vi "ReadSensorValues_v1.1.vi"(10 "VISA resource name":refnum<visa-resource-name>, 11 "Sensor type":T1) -> ()   [LabVIEW 2012]
uses:
  <vilib>/nican/nicantsk.llb/CAN Interface.ctl
  SensorTypes.ctl
  SensorStates.ctl
  <vilib>/nican/nicantsk.llb/CAN Task Reference.ctl
  <vilib>/nican/nicantsk.llb/CAN Mode.ctl
  globalVariables.vi
  <vilib>/nican/nicantsk.llb/CAN Read Multi Chan Single Samp 1D Dbl.vi
  <instrlib>/Agilent 34970/Agilent 34970.lvlib
panel:
  in  "Sample time reference sensor / s":dbl=0.05
  in  "VISA resource name 2":refnum<visa-resource-name>="USB0::0x0957::0x2007::MY49004365::INSTR"
  in  "Cancel Measurement":bool
  out "new data":bool
  out "running":bool
  out "Sample number":i32
  in  "Interface":T2 items=["CAN0"=0, "CAN1"=1, "CAN2"=2, "CAN3"=3, "CAN4"=4, "CAN5"=5, "CAN6"=6, "CAN7"=7, "CAN8"=8, "CAN9"=9, "CAN10"=10, "CAN11"=11, "CAN12"=12, "CAN13"=13, "CAN14"=14, "CAN15"=15, "CAN16"=16, "CAN17"=17, "CAN18"=18, "CAN19"=19, "CAN20"=20, "CAN21"=21, "CAN22"=22, "CAN23"=23, "CAN24"=24, "CAN25"=25, "CAN26"=26, "CAN27"=27, "CAN28"=28, "CAN29"=29, "CAN30"=30, "CAN31"=31, "CAN32"=32, "CAN33"=33, "CAN34"=34, "CAN35"=35, "CAN36"=36, "CAN37"=37, "CAN38"=38, "CAN39"=39, "CAN40"=40, "CAN41"=41, "CAN42"=42, "CAN43"=43, "CAN44"=44, "CAN45"=45, "CAN46"=46, "CAN47"=47, "CAN48"=48, "CAN49"=49, "CAN50"=50, "CAN51"=51, "CAN52"=52, "CAN53"=53, "CAN54"=54, "CAN55"=55, "CAN56"=56, "CAN57"=57, "CAN58"=58, "CAN59"=59, "CAN60"=60, "CAN61"=61, "CAN62"=62, "CAN63"=63, "MAX default"=64, "CAN256 (Virtual)"=256, "CAN257 (Virtual)"=257]
  out "Error Flag":bool
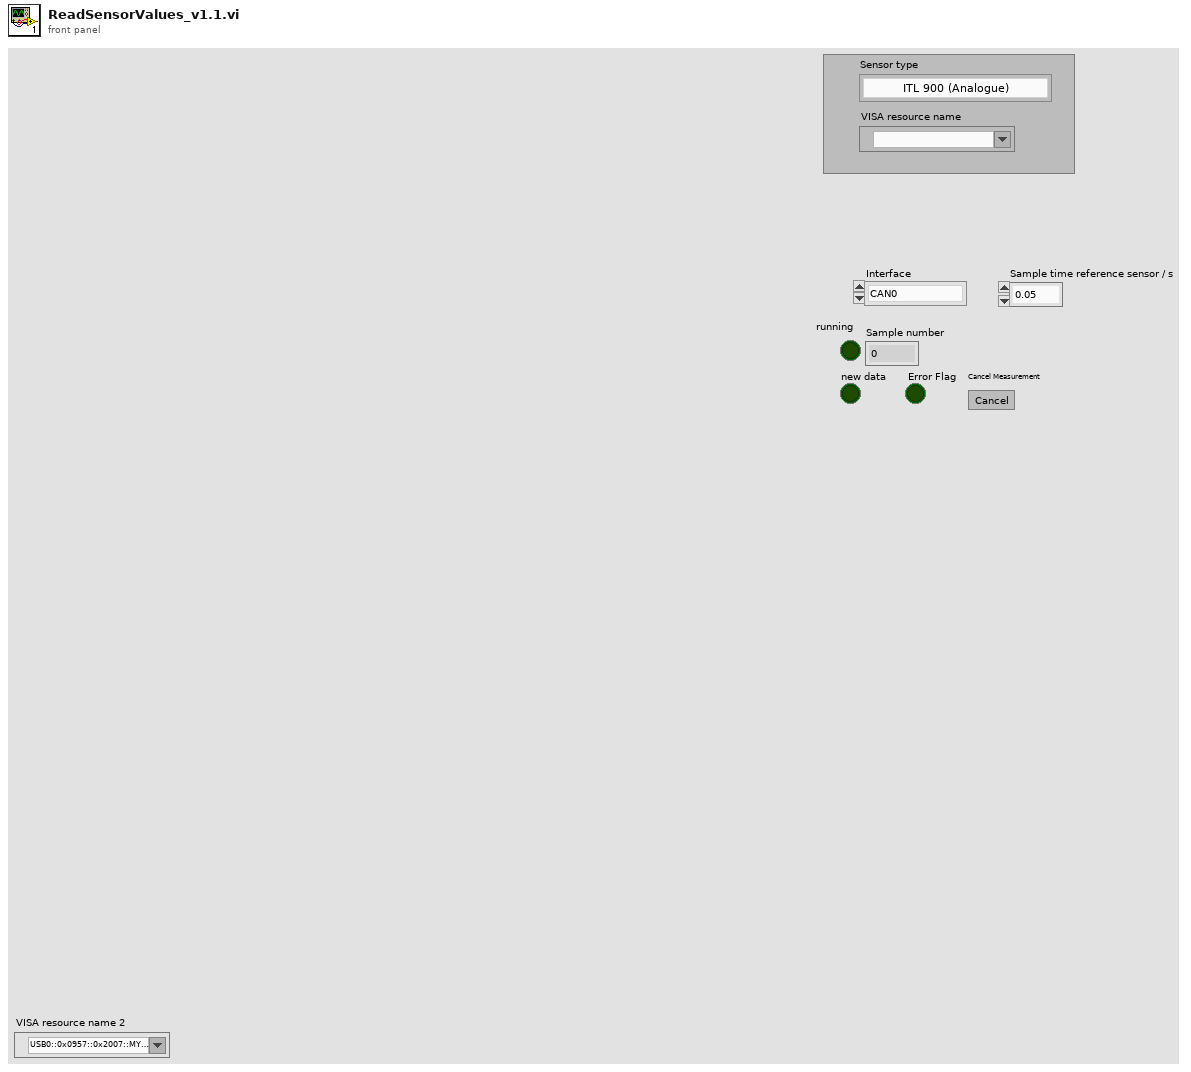
[diagram p1: front panel]
types:
  T1 = typedef "SensorTypes.ctl" = enum16{"ITL 900 (Analogue)", "CAB 300-C SP3 (CAN)", "xyz TODO (PWM)", "xyz TODO (LIN)", "xyz TODO (Analogue)"}
  T2 = typedef "CAN Interface.ctl" = u16
  T3 = typedef "SensorStates.ctl" = enum16{"init", "measure", "terminate"}
  T4 = cluster{"Include Alarm Data F:(No)":bool, "Include Channel # (F:No)":bool, "Include Time (F:No)":bool, "Include Units (F:No)":bool}
  T5 = cluster{"Aperture Value (.4)":dbl, "Aperture (1:Minimum)":u16, "NPLC (1)":u16, "Bandwidth (3 Hz)":u16, "Input Impedance (F:Fixed)":bool, "Integration Time (F:Aperture)":bool}
  T6 = enum16{"100 mV", "1 V", "10 V", "100 V", "300 V", "Minimum", "Maximum"}
  T7 = enum16{"Manual", "Minimum", "Maximum", "Infinity"}
  T8 = enum16{"Bus", "Immediate", "External", "Alarm 1", "Alarm 2", "Alarm 3", "Alarm 4", "Timer"}
  T9 = cluster{"Timeout Value (10000)":u32, "Baud Rate (57600)":enum16{"1200", "2400", "4800", "9600", "19200", "38400", "57600", "115200"}, "Flow Control (1:XON/XOFF)":enum16{"None", "XON / XOFF", "RTS / CTS", "DTR / DSR"}}
  T10 = typedef "CAN Task Reference.ctl" = u32
  T11 = enum16{"Remote Trigger", "Immediate Trigger", "Wait for Trigger", "Abort Scan"}
  T12 = typedef "CAN Mode.ctl" = u16
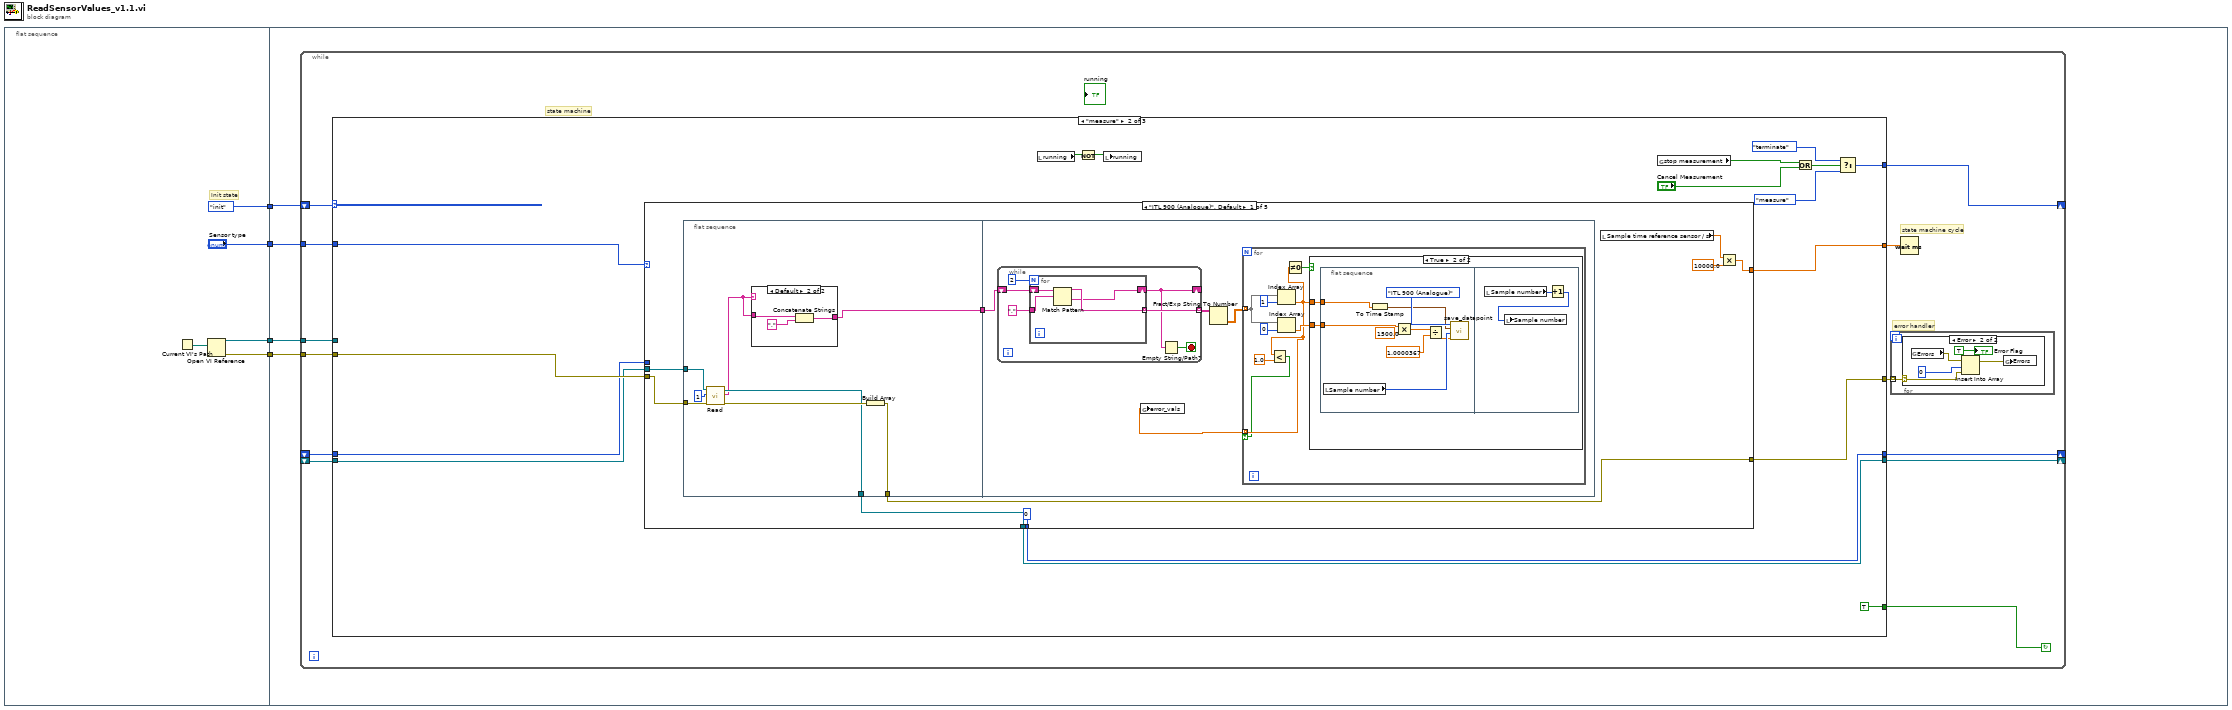
[diagram p0: block diagram]
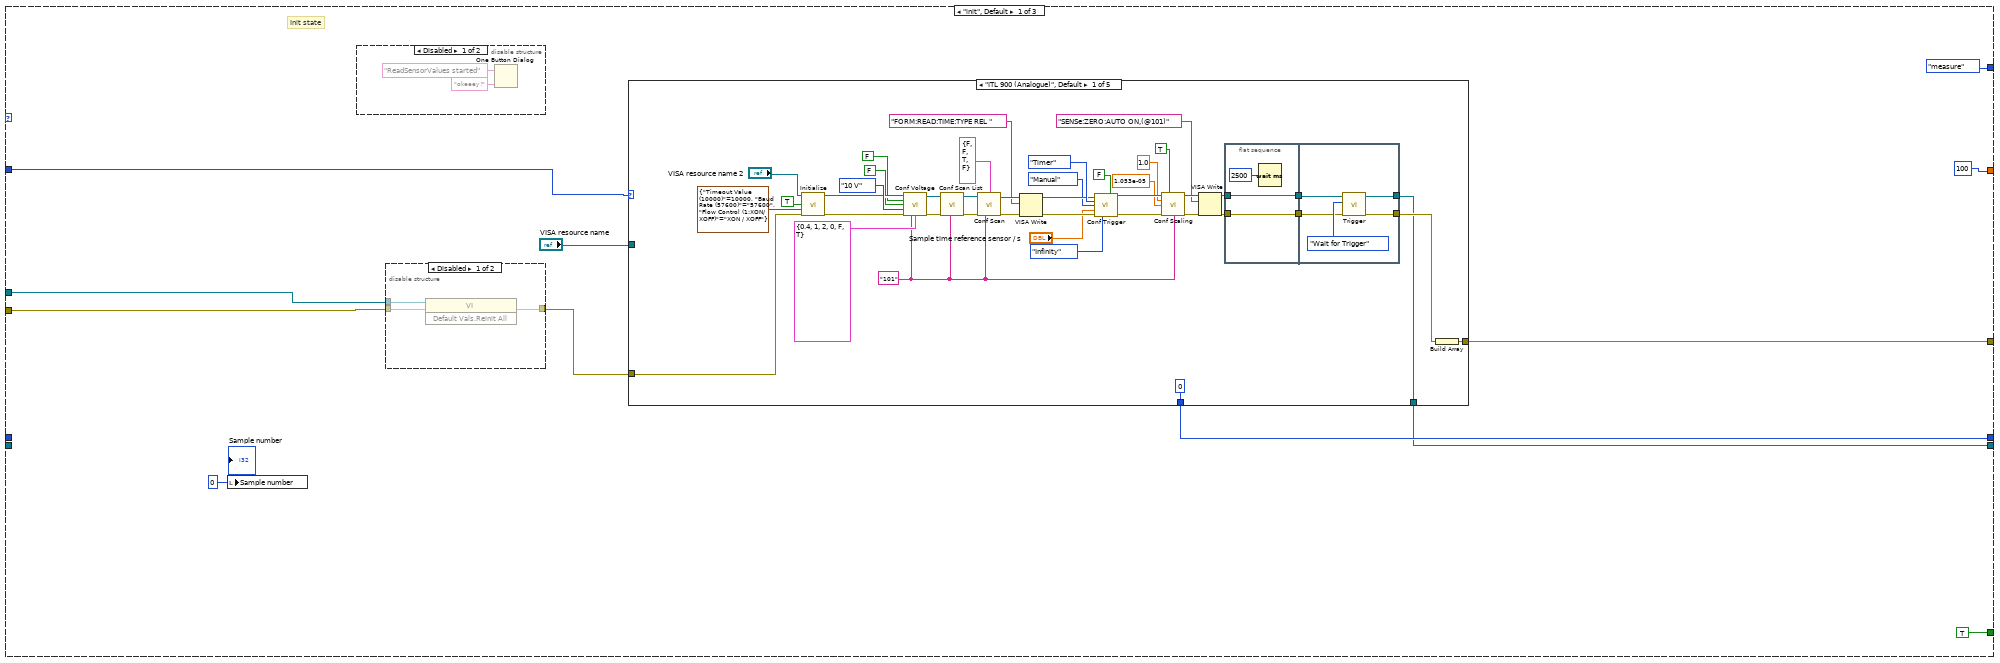
[diagram p3: hidden frame]
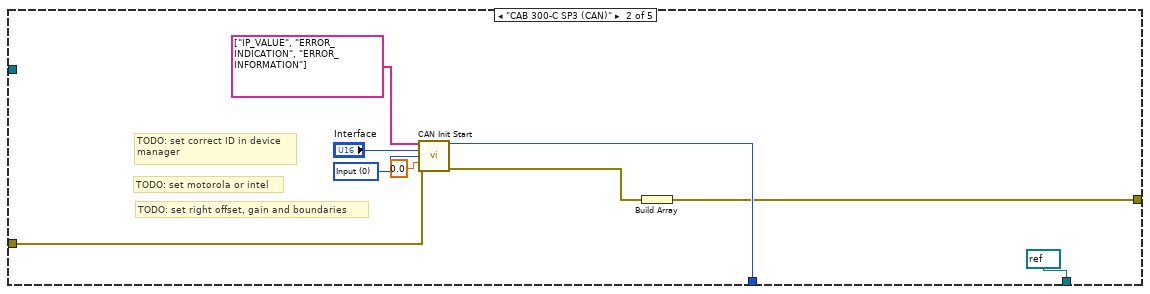
[diagram p6: hidden frame]
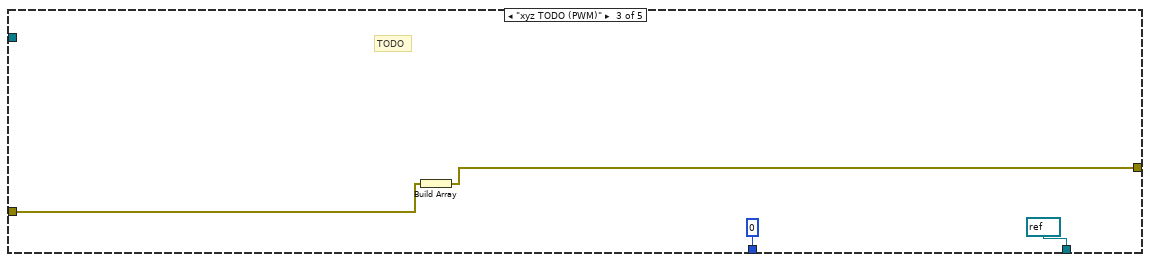
[diagram p7: hidden frame]
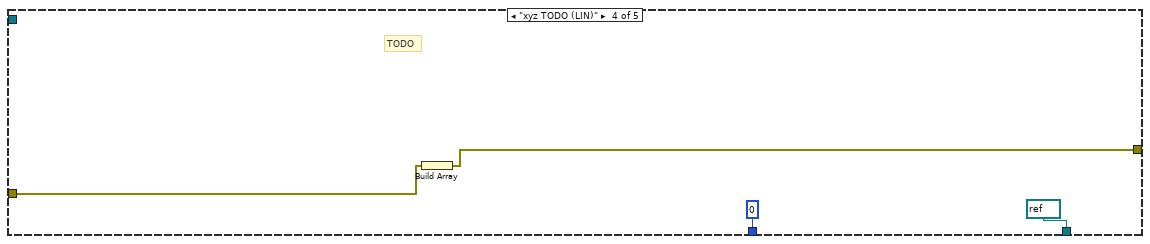
[diagram p8: hidden frame]
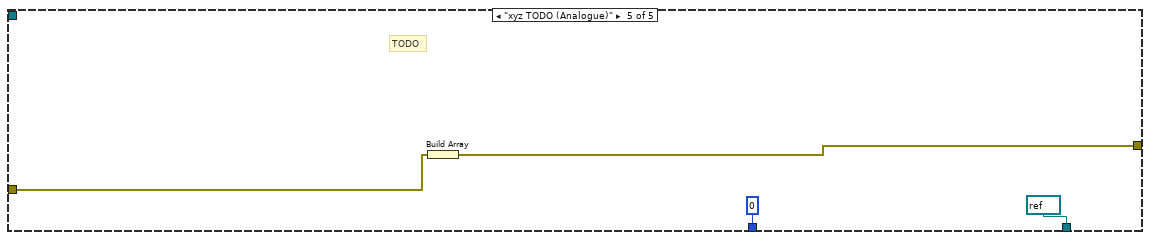
[diagram p9: hidden frame]
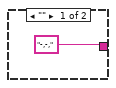
[diagram p10: hidden frame]
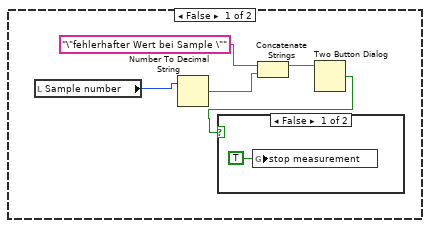
[diagram p11: hidden frame]
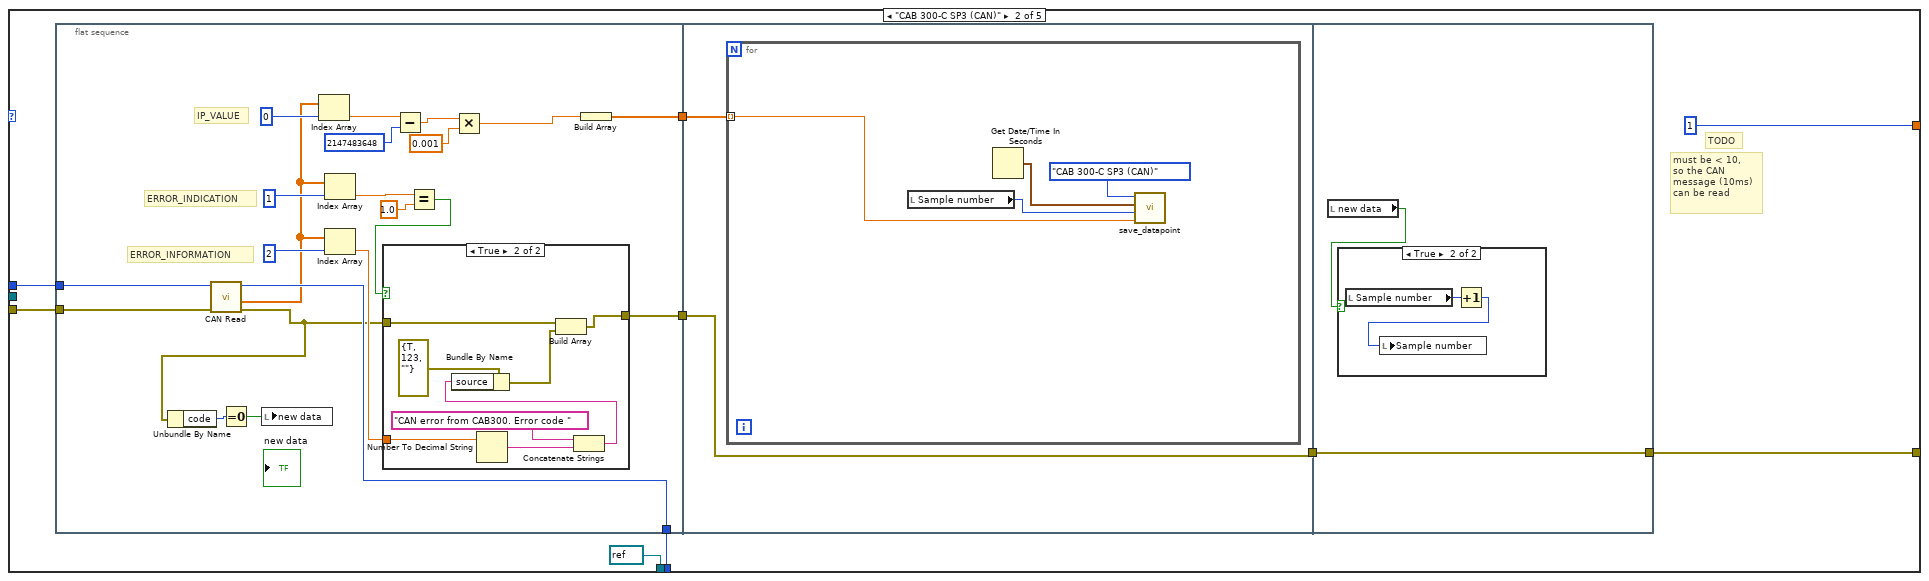
[diagram p13: hidden frame]
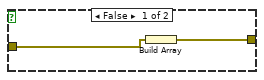
[diagram p14: hidden frame]
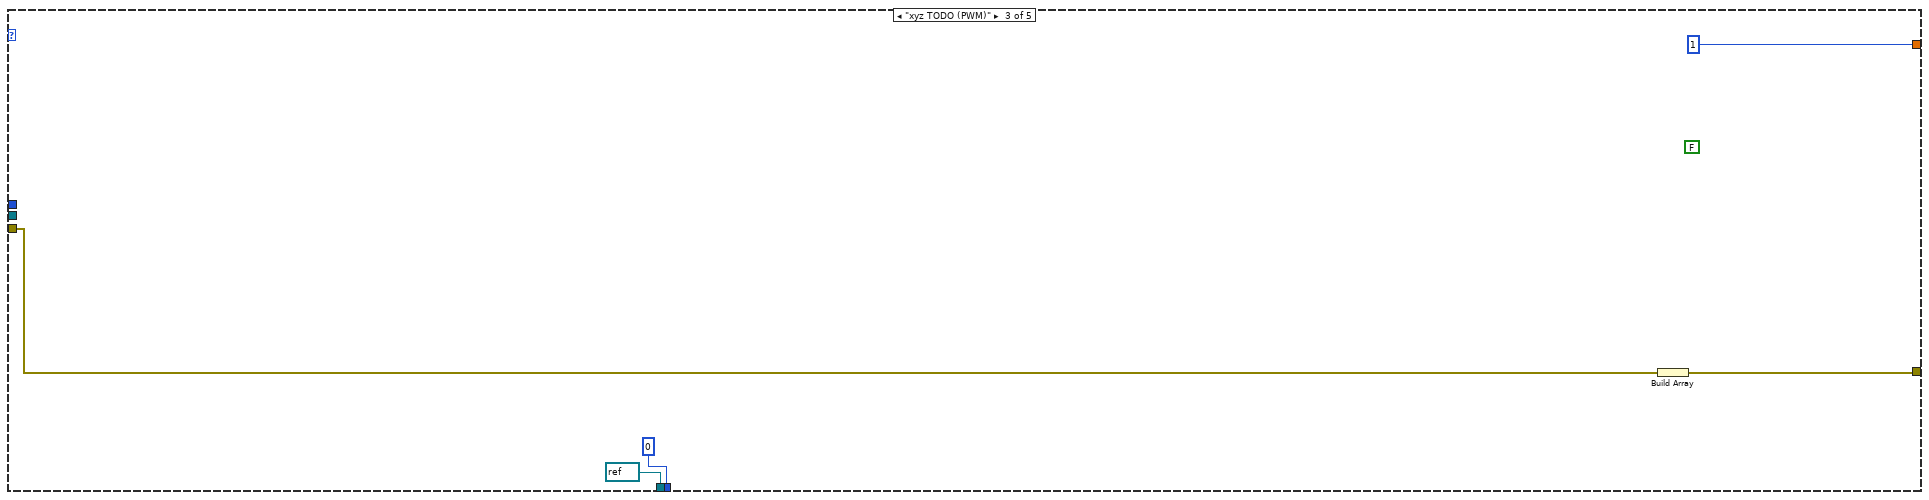
[diagram p16: hidden frame]
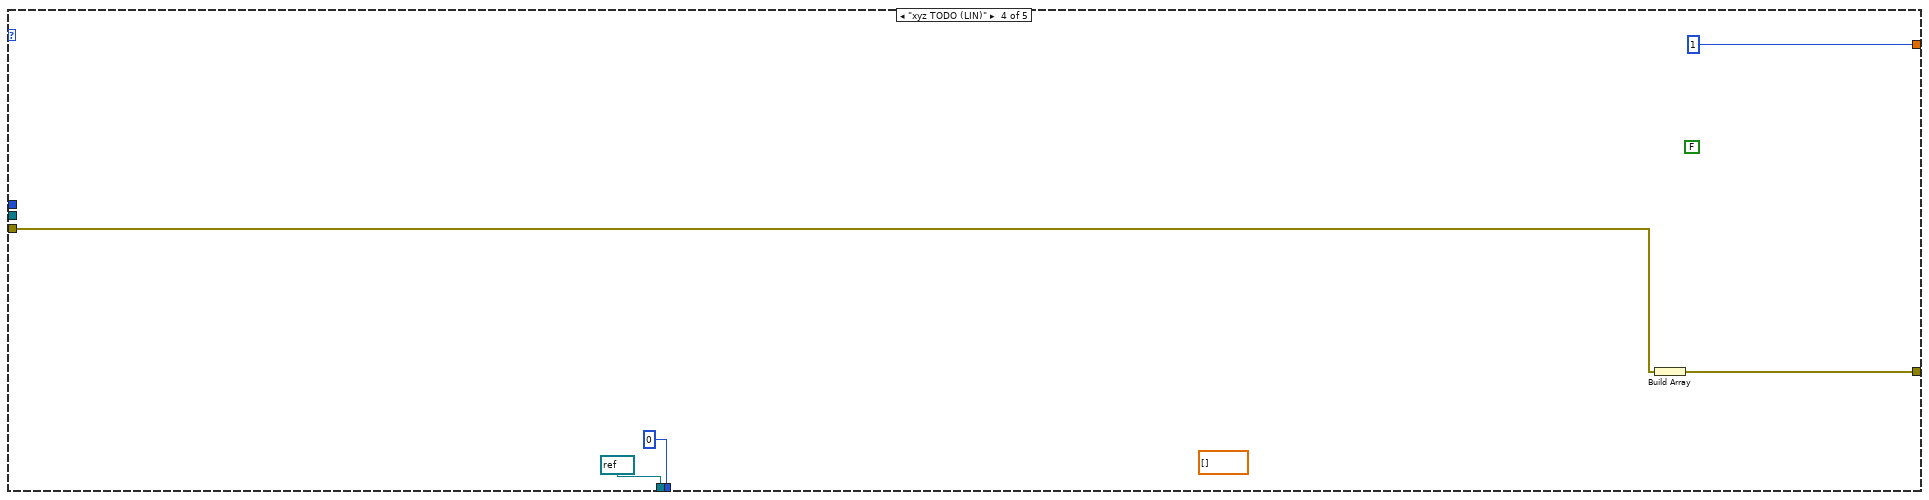
[diagram p17: hidden frame]
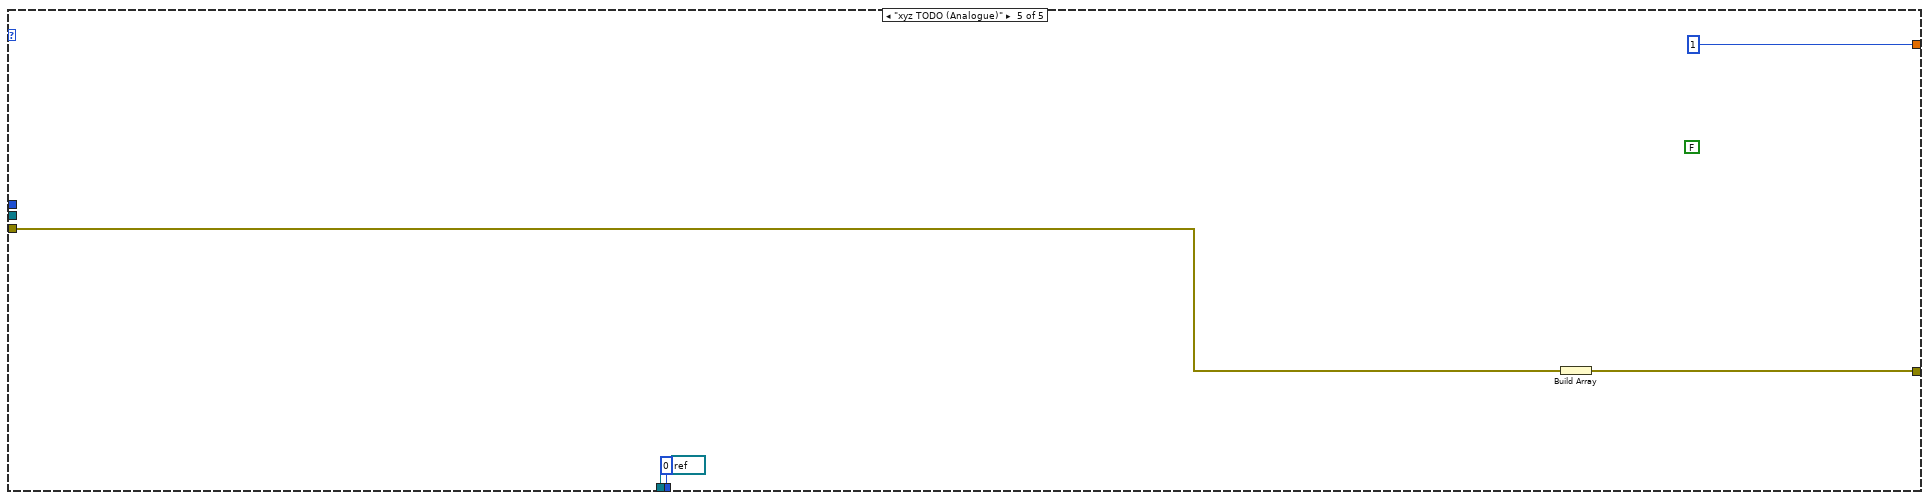
[diagram p18: hidden frame]
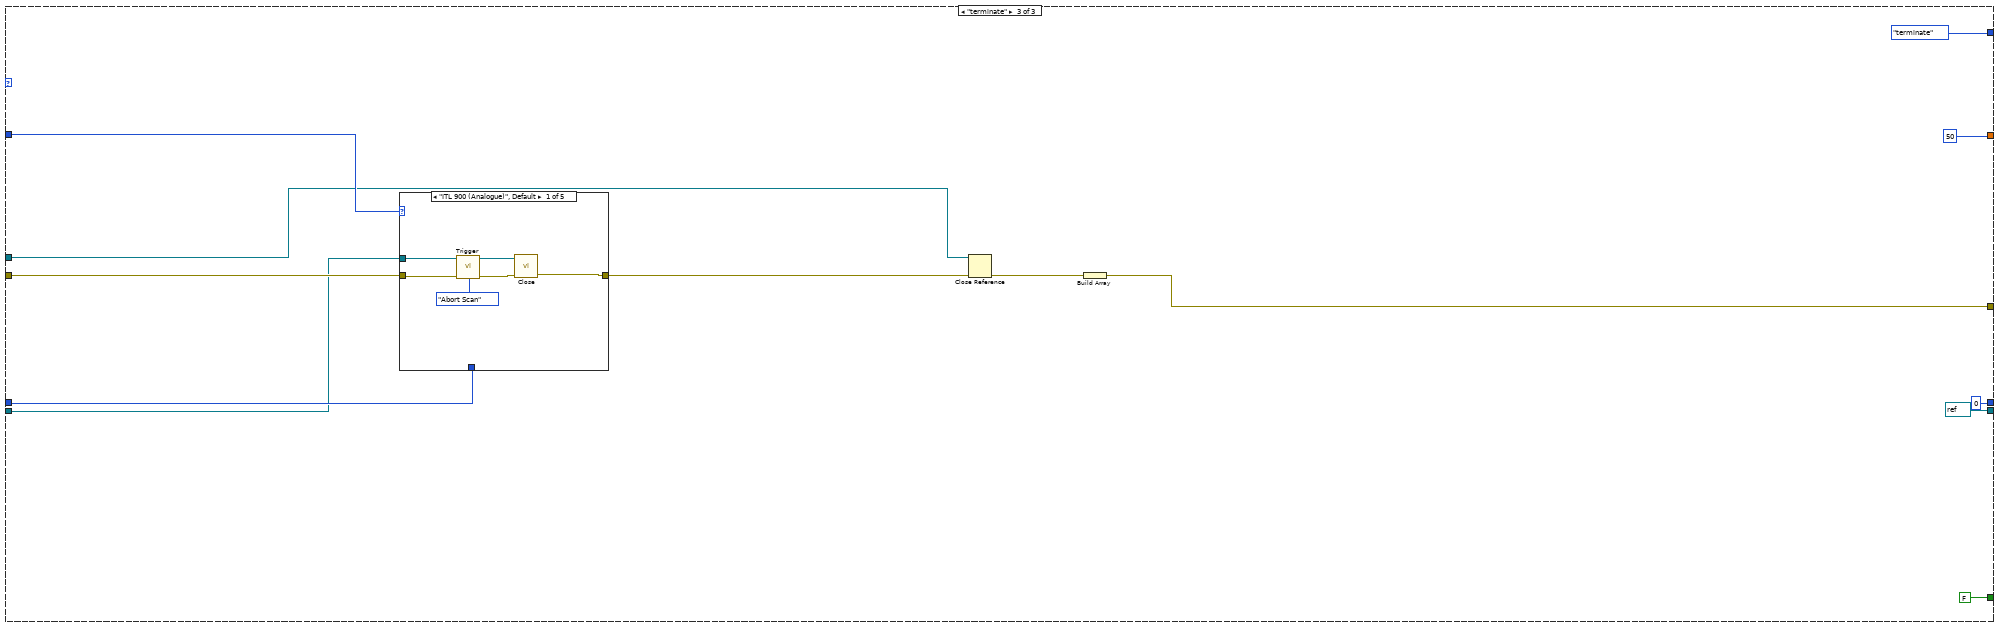
[diagram p19: hidden frame]
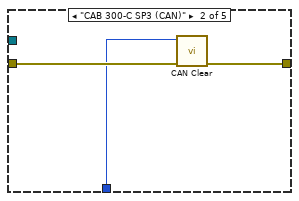
[diagram p20: hidden frame]
diagram:
  n1 = flat-sequence {
    tunnel: [SensorStates."init" ("States IEEE-488")] -> w4
    tunnel: [w9] -> w3
    tunnel: [w8] -> w2
    tunnel: ["Sensor type"] -> w1
    tunnel: w4 -> [w11]
    tunnel: w3 -> [w13]
    tunnel: w2 -> [w12]
    tunnel: w1 -> [w10]
    frame #0 {
      # "Init state"
      n2 = Current VI's Path() -> (path=w7:path)
      n3 = Open VI Reference(vi path=w7) -> (vi reference=w9:refnum<vi>, error out=w8:errorcluster)  [unwired: 2 in, 3 out]
    }
    frame #1 {
      n4 = while {
        tunnel: w13 -> [w24]
        tunnel: w12 -> [w23]
        shift-right: [w21] -> _
        shift-left: w11 -> [w22]
        shift-right: [w20] -> _
        shift-left: _ -> [w19]
        tunnel: w10 -> [w17]
        shift-right: [w15] -> _
        shift-left: _ -> [w14]
        stop <- w16 continue-if-true
        # "state machine"
        # "error handler"
        # "state machine cycle"
        n5 = case shown="\"measure\"" w22 {
          tunnel: [u32 100 ("milliseconds to wait") w120 u32 50 ("milliseconds to wait")] -> w25
          tunnel: w24 -> [w41 _ w268]
          tunnel: w23 -> [w42 w133 w273]
          tunnel: [SensorStates."measure" ("States IEEE-488") w134 SensorStates."terminate" ("States IEEE-488")] -> w21
          tunnel: [w39 w127 T10 0 ("task reference out")] -> w20
          tunnel: w19 -> [_ w128 w272]
          tunnel: [w37 w129 w271] -> w18
          tunnel: w17 -> [w35 w121 w270]
          tunnel: [TRUE TRUE FALSE] -> w16
          tunnel: [w32 w122 refnum<visa-resource-name> refnum ("VISA Resource Name Out")] -> w15
          tunnel: w14 -> [_ w123 w265]
          frame "init", Default {
            # "Init state"
            n6 = local write "Sample number"(0 ("Sample number")) -> ()
            n7 = disable-structure shown="Disabled" {
              frame Disabled {
                n8 = One Button Dialog(message="ReadSensorValues started", button name ("OK")="okeeey!") -> ()  [unwired: 1 out]
              }
              frame Enabled {
              }
            }
            n9 = disable-structure shown="Disabled" {
              disable-tunnel: w42 -> [w46 _]
              disable-tunnel: w41 -> [w45 _]
              disable-tunnel: [w44 _] -> w38
              frame Disabled {
                n10 = invoke class="VI" method="Default Vals.Reinit All"(reference=w45, error in=w46) -> (error out=w44:errorcluster)  [unwired: 1 in, 2 out]
              }
              frame Enabled {
              }
            }
            n11 = case shown="\"ITL 900 (Analogue)\", Default" w35 {
              tunnel: [T10 0 ("task reference out") w103 T10 0 ("task reference out") T10 0 ("task reference out") T10 0 ("task reference out")] -> w39
              tunnel: w38 -> [w52 w102 w110 w114 w119]
              tunnel: [w90 w100 w111 w115 w118] -> w37
              tunnel: "VISA resource name" -> [_ _ _ _ _]
              tunnel: [w50 refnum<visa-resource-name> refnum ("VISA Resource Name Out") refnum<visa-resource-name> refnum ("VISA Resource Name Out") refnum<visa-resource-name> refnum ("VISA Resource Name Out") refnum<visa-resource-name> refnum ("VISA Resource Name Out")] -> w32
              frame "ITL 900 (Analogue)", Default {
                w59 = "101" ("Channel List (Volt.)")
                n12 = call <instrlib>:"Initialize.vi"("VISA Resource Name"="VISA resource name 2", "Reset (T: Reset)"=TRUE, "Serial Port Configuration"=T9 {"Timeout Value (10000)"=10000, "Baud Rate (57600)"=enum."57600", "Flow Control (1:XON/XOFF)"=enum."XON / XOFF"}, "error in (no error)"=w52) -> ("VISA Resource Name Out"=w84:refnum<visa-resource-name>, "error out"=w80:errorcluster)  [unwired: 10 in]
                n13 = call <instrlib>:"Conf Voltage.vi"("VISA Resource Name"=w84, "AC/DC (F:DC)"=FALSE, "Autorange? (F:Off)"=FALSE, "Range (6:Max)"=T6."10 V" ("Range (Volt.)"), "error in (no error)"=w80, "Channel List (empty)"=w59, "Advanced Config"=T5 {"Aperture Value (.4)"=0.4, "Aperture (1:Minimum)"=1, "NPLC (1)"=2, "Bandwidth (3 Hz)"=0, "Input Impedance (F:Fixed)"=FALSE, "Integration Time (F:Aperture)"=TRUE}) -> ("VISA Resource Name Out"=w82:refnum<visa-resource-name>, "error out"=w77:errorcluster)  [unwired: 6 in, 1 out]
                n14 = call <instrlib>:"Conf Scan List.vi"("Scan List (empty)"=w59, "error in (no error)"=w77, "VISA Resource Name"=w82) -> ("error out"=w76:errorcluster, "VISA Resource Name Out"=w78:refnum<visa-resource-name>)  [unwired: 6 in, 1 out]
                n15 = call <instrlib>:"Conf Scan.vi"("VISA Resource Name"=w78, "error in (no error)"=w76, "Channel List (empty)"=w59, "Scan Fields"=T4 {"Include Alarm Data F:(No)"=FALSE, "Include Channel # (F:No)"=FALSE, "Include Time (F:No)"=TRUE, "Include Units (F:No)"=FALSE}) -> ("VISA Resource Name Out"=w72:refnum<visa-resource-name>, "error out"=w71:errorcluster)  [unwired: 9 in, 1 out]
                n16 = VISA Write(VISA resource name=w72, write buffer="FORM:READ:TIME:TYPE REL ", error in (no error)=w71) -> (VISA resource name out=w69:refnum<visa-resource-name>, error out=w70:errorcluster)  [unwired: 1 out]
                n17 = call <instrlib>:"Conf Trigger.vi"("VISA Resource Name"=w69, "Wait for Trigger? (F:No)"=FALSE, "Source (1:Immediate)"=T8."Timer", "Time-Scan Interval (1:Min)"=enum16{"Manual", "Minimum", "Maximum"}."Manual", "Interval Value (0)"="Sample time reference sensor / s", "error in (no error)"=w70, "Max Trigger Count (3:Inf)"=T7."Infinity") -> ("VISA Resource Name Out"=w63:refnum<visa-resource-name>, "error out"=w62:errorcluster)  [unwired: 6 in, 1 out]
                n18 = call <instrlib>:"Conf Scaling.vi"("VISA Resource Name"=w63, "Enable Scaling? (T:Enable)"=TRUE, "Gain (1)"=1.0, "Offset (0)"=1.053e-05, "error in (no error)"=w62, "Channel List (empty)"=w59) -> ("VISA Resource Name Out"=w58:refnum<visa-resource-name>, "error out"=w57:errorcluster)  [unwired: 7 in, 1 out]
                n19 = VISA Write(VISA resource name=w58, write buffer="SENSe:ZERO:AUTO ON,(@101)", error in (no error)=w57) -> (VISA resource name out=w55:refnum<visa-resource-name>, error out=w54:errorcluster)  [unwired: 1 out]
                n20 = flat-sequence {
                  tunnel: [w92] -> w88
                  tunnel: w55 -> [w92]
                  tunnel: [w91] -> w87
                  tunnel: w54 -> [w91]
                  tunnel: [w98] -> w50
                  tunnel: [w97] -> w51
                  tunnel: w88 -> [w95]
                  tunnel: w87 -> [w94]
                  frame #0 {
                    n21 = Wait (ms)(milliseconds to wait=u32 2500) -> ()  [unwired: 1 out]
                  }
                  frame #1 {
                    n22 = call <instrlib>:"Trigger.vi"("error in (no error)"=w94, "Command (0:Rem Trig)"=T11."Wait for Trigger", "VISA Resource Name"=w95) -> ("error out"=w97:errorcluster, "VISA Resource Name Out"=w98:refnum<visa-resource-name>)  [unwired: 7 in]
                  }
                }
                n23 = Build Array(w51) -> (w90:errorcluster[])
              }
              frame "CAB 300-C SP3 (CAN)" {
                w104 = T12 0 items=["Input", "Output", "Timestamped Input", "Output Recent"] ("mode")
                # "TODO: set right offset, gain and boundaries"
                # "TODO: set motorola or intel"
                # "TODO: set correct ID in device\nmanager"
                n24 = call <vilib>:"CAN Init Start.vi"("channel list"=string[] ["IP_VALUE", "ERROR_INDICATION", "ERROR_INFORMATION"] ("Channel List"), "interface"="Interface", "mode"=w104, "sample rate"=0.0, "error in (no error)"=w102) -> ("task reference out"=w103:T10, "error out"=w101:errorcluster)  [unwired: 9 in]
                n25 = Build Array(w101) -> (w100:errorcluster[])
              }
              frame "xyz TODO (PWM)" {
                # "TODO"
                n26 = Build Array(w110) -> (w111:errorcluster[])
              }
              frame "xyz TODO (LIN)" {
                # "TODO"
                n27 = Build Array(w114) -> (w115:errorcluster[])
              }
              frame "xyz TODO (Analogue)" {
                # "TODO"
                n28 = Build Array(w119) -> (w118:errorcluster[])
              }
            }
          }
          frame "measure" {
            n29 = case shown="\"ITL 900 (Analogue)\", Default" w121 {
              tunnel: w133 -> [w144 w204 w252 w256 w261]
              tunnel: [w141 w203 w253 w257 w262] -> w129
              tunnel: w128 -> [_ w202 _ _ _]
              tunnel: [T10 0 ("task reference out") w201 T10 0 ("task reference out") T10 0 ("task reference out") T10 0 ("task reference out")] -> w127
              tunnel: w123 -> [w145 _ _ _ _]
              tunnel: [w142 refnum<visa-resource-name> refnum ("VISA Resource Name Out") refnum<visa-resource-name> refnum ("VISA Resource Name Out") refnum<visa-resource-name> refnum ("VISA Resource Name Out") refnum<visa-resource-name> refnum ("VISA Resource Name Out")] -> w122
              tunnel: [w137 u32 1 ("milliseconds to wait") u32 1 ("milliseconds to wait") u32 1 ("milliseconds to wait") u32 1 ("milliseconds to wait")] -> w120
              frame "ITL 900 (Analogue)", Default {
                n30 = flat-sequence {
                  tunnel: w145 -> [w151]
                  tunnel: w144 -> [w150]
                  tunnel: [w149] -> w143
                  tunnel: [w148] -> w142
                  tunnel: [w147] -> w141
                  tunnel: w143 -> [w161]
                  frame #0 {
                    n31 = call <instrlib>:"Read.vi"("error in (no error)"=w150, "# Channels (1)"=1, "VISA Resource Name"=w151) -> ("error out"=w152:errorcluster, "Readings"=w146:string, "VISA Resource Name Out"=w148:refnum<visa-resource-name>)  [unwired: 5 in, 1 out]
                    n32 = case shown="Default" w146 {
                      tunnel: ["-,-," ("string") w157] -> w149
                      tunnel: w146 -> [_ w156]
                      frame "" {
                      }
                      frame Default {
                        n33 = Concatenate Strings(w156, "," ("string")) -> (w157:string)
                      }
                    }
                    n34 = Build Array(w152) -> (w147:errorcluster[])
                  }
                  frame #1 {
                    n35 = while {
                      tunnel: [w166] -> w160 mode=indexing
                      shift-left: w161 -> [w167]
                      shift-right: [w163] -> _
                      stop <- w165 stop-if-true
                      n36 = for {
                        N: 2 -> [_]
                        tunnel: [w169] -> w166 mode=indexing
                        tunnel: "," ("regular expression") -> [w170]
                        shift-right: [w168] -> w163
                        shift-left: w167 -> [w171]
                        n37 = Match Pattern(string=w171, regular expression=w170) -> (before substring=w169:string, after substring=w168:string)  [unwired: 1 in, 2 out]
                      }
                      n38 = Empty String/Path?(string/path=w163) -> (empty?=w165:bool)
                    }
                    n39 = Fract/Exp String To Number(string=w160) -> (number=w159:dbl[][])  [unwired: 3 in, 1 out]
                    n40 = for {
                      tunnel: w159 -> [w177] mode=indexing
                      tunnel: [w173] -> w158 mode=indexing if=w172
                      n41 = Index Array(array=w177, index=1 ("disabled index (col)")) -> (element=w173:dbl)
                      n42 = Less?(x=w173, y=1.0) -> (x < y?=w172:bool)
                      n43 = Index Array(array=w177, index=0 ("disabled index (col)")) -> (element=w176:dbl)
                      n44 = Not Equal To 0?(x=w173) -> (x != 0?=w175:bool)
                      n45 = case shown="True" w175 {
                        tunnel: w173 -> [_ w187]
                        tunnel: w176 -> [_ w186]
                        frame False {
                          n46 = local read "Sample number"() -> (w184:i32)
                          n47 = Number To Decimal String(number=w184) -> (decimal integer string=w181:string)  [unwired: 1 in]
                          n48 = Concatenate Strings("\"fehlerhafter Wert bei Sample \"" ("message"), w181) -> (w183:string)
                          n49 = Two Button Dialog(message=w183) -> (T button?=w180:bool)  [unwired: 2 in]
                          n50 = case shown="False" w180 {
                            frame False {
                              n51 = global write "globalVariables.vi" "stop measurement"(TRUE ("stop measurement")) -> ()
                            }
                            frame True {
                            }
                          }
                        }
                        frame True {
                          n52 = flat-sequence {
                            tunnel: w187 -> [w189]
                            tunnel: w186 -> [w188]
                            frame #0 {
                              n53 = local read "Sample number"() -> (w195:i32)
                              n54 = To Time Stamp(1:w189) -> (0:w190:timestamp)
                              n55 = Multiply(x=w188, y=1500.0) -> (x*y=w192:dbl)
                              n56 = Divide(x=w192, y=1.0000367) -> (x/y=w191:dbl)
                              n57 = call "save_datapoint.vi"("current value"=w191, "Sample number"=w195, "current time of measurement"=w190, "Sensor type"=SensorTypes."ITL 900 (Analogue)") -> ()
                            }
                            frame #1 {
                              n58 = local read "Sample number"() -> (w198:i32)
                              n59 = Increment(x=w198) -> (x+1=w197:i32)
                              n60 = local write "Sample number"(w197) -> ()
                            }
                          }
                        }
                      }
                    }
                    n61 = global write "globalVariables.vi" "error_vals"(w158) -> ()
                  }
                }
                n62 = local read "Sample time reference sensor / s"() -> (w139:dbl)
                n63 = Multiply(x=w139, y=10000.0) -> (x*y=w137:dbl)
              }
              frame "CAB 300-C SP3 (CAN)" {
                # "TODO"
                # "must be < 10,\nso the CAN \nmessage (10ms) \ncan be read"
                n64 = flat-sequence {
                  tunnel: [w227] -> w207
                  tunnel: [w226] -> w206
                  tunnel: w204 -> [w228]
                  tunnel: w202 -> [w225]
                  tunnel: [w224] -> w201
                  tunnel: w207 -> [w240]
                  tunnel: w206 -> [w239]
                  tunnel: [w240] -> w205
                  tunnel: w205 -> [w246]
                  tunnel: [w246] -> w203
                  frame #0 {
                    # "ERROR_INFORMATION"
                    # "ERROR_INDICATION"
                    # "IP_VALUE"
                    n65 = call-poly <vilib>:"CAN Read.vi"("error in (no error)"=w228, "task reference in"=w225) -> ("error out"=w215:errorcluster, "multi-chan single-samp 1D dbl"=w218:dbl[], "task reference out"=w224:T10)  [unwired: 6 in, 1 out]
                    n66 = Unbundle By Name(w215) -> ("code"=w214:i32)
                    n67 = Equal To 0?(x=w214) -> (x = 0?=w213:bool)
                    n68 = local write "new data"(w213) -> ()
                    n69 = Index Array(array=w218, index=0) -> (element=w212:dbl)
                    n70 = Index Array(array=w218, index=1) -> (element=w220:dbl)
                    n71 = Index Array(array=w218, index=2) -> (element=w217:dbl)
                    n72 = Subtract(x=w212, y=u32 2147483648) -> (x-y=w210:dbl)
                    n73 = Equal?(x=w220, y=1.0) -> (x = y?=w216:bool)
                    n74 = case shown="True" w216 {
                      tunnel: w215 -> [w230 w238]
                      tunnel: [w229 w237] -> w227
                      tunnel: w217 -> [_ w232]
                      frame False {
                        n75 = Build Array(w230) -> (w229:errorcluster[])
                      }
                      frame True {
                        n76 = Number To Decimal String(number=w232) -> (decimal integer string=w233:string)  [unwired: 1 in]
                        n77 = Concatenate Strings("CAN error from CAB300. Error code ", w233) -> (w231:string)
                        n78 = Bundle By Name(cluster=errorcluster {"status"=TRUE, "code"=123, "source"=""} ("error out"), "source"=w231) -> (w235:errorcluster)
                        n79 = Build Array(w238, w235) -> (w237:errorcluster[])
                      }
                    }
                    n80 = Multiply(x=w210, y=0.001) -> (x*y=w208:dbl)
                    n81 = Build Array(w208) -> (w226:dbl[])
                  }
                  frame #1 {
                    n82 = for {
                      tunnel: w239 -> [w242] mode=indexing
                      n83 = local read "Sample number"() -> (w244:i32)
                      n84 = Get Date/Time In Seconds() -> (seconds since 1Jan1904=w241:timestamp)
                      n85 = call "save_datapoint.vi"("current value"=w242, "Sample number"=w244, "current time of measurement"=w241, "Sensor type"=SensorTypes."CAB 300-C SP3 (CAN)") -> ()
                    }
                  }
                  frame #2 {
                    n86 = local read "new data"() -> (w245:bool)
                    n87 = case shown="True" w245 {
                      frame False {
                      }
                      frame True {
                        n88 = local read "Sample number"() -> (w248:i32)
                        n89 = Increment(x=w248) -> (x+1=w247:i32)
                        n90 = local write "Sample number"(w247) -> ()
                      }
                    }
                  }
                }
              }
              frame "xyz TODO (PWM)" {
                (unwired) FALSE ("new data")
                n91 = Build Array(w252) -> (w253:errorcluster[])
              }
              frame "xyz TODO (LIN)" {
                (unwired) dbl[] []
                (unwired) FALSE ("new data")
                n92 = Build Array(w256) -> (w257:errorcluster[])
              }
              frame "xyz TODO (Analogue)" {
                (unwired) FALSE ("new data")
                n93 = Build Array(w261) -> (w262:errorcluster[])
              }
            }
            n94 = local read "running"() -> (w131:bool)
            n95 = Not(x=w131) -> (.not. x?=w132:bool)
            n96 = local write "running"(w132) -> ()
            n97 = global read "globalVariables.vi" "stop measurement"() -> (w126:bool)
            n98 = Or(x=w126, y="Cancel Measurement") -> (x .or. y?=w124:bool)
            n99 = Select(t=SensorStates."terminate" ("States IEEE-488"), s=w124, f=SensorStates."measure" ("States IEEE-488")) -> (s? t:f=w134:T3)
          }
          frame "terminate" {
            n100 = case shown="\"ITL 900 (Analogue)\", Default" w270 {
              tunnel: w273 -> [w279 w285 w286 w287 w288]
              tunnel: [w278 w284 w286 w287 w288] -> w267
              tunnel: w272 -> [_ w283 _ _ _]
              tunnel: w265 -> [w277 _ _ _ _]
              frame "ITL 900 (Analogue)", Default {
                n101 = call <instrlib>:"Trigger.vi"("error in (no error)"=w279, "Command (0:Rem Trig)"=T11."Abort Scan", "VISA Resource Name"=w277) -> ("error out"=w281:errorcluster, "VISA Resource Name Out"=w280:refnum<visa-resource-name>)  [unwired: 7 in]
                n102 = call <instrlib>:"Close.vi"("VISA Resource Name"=w280, "error in (no error)"=w281) -> ("error out"=w278:errorcluster)  [unwired: 13 in]
              }
              frame "CAB 300-C SP3 (CAN)" {
                n103 = call <vilib>:"CAN Clear.vi"("error in (no error)"=w285, "task reference in"=w283) -> ("error out"=w284:errorcluster)  [unwired: 9 in]
              }
              frame "xyz TODO (PWM)" {
              }
              frame "xyz TODO (LIN)" {
              }
              frame "xyz TODO (Analogue)" {
              }
            }
            n104 = Close Reference(reference=w268, error in (no error)=w267) -> (error out=w275:errorcluster)
            n105 = Build Array(w275) -> (w271:errorcluster[])
          }
        }
        n106 = for {
          tunnel: w18 -> [w26] mode=indexing
          n107 = case shown="Error" w26 {
            selector: w26 -> [_ w30]
            frame No Error {
            }
            frame Error {
              n108 = global read "globalVariables.vi" "Errors"() -> (w28:errorcluster[])
              n109 = Insert Into Array(array=w28, index=0, new element=w30) -> (w27:errorcluster[])
              n110 = global write "globalVariables.vi" "Errors"(w27) -> ()
              "Error Flag" <- TRUE ("Error Flag")
            }
          }
        }
        n111 = Wait (ms)(milliseconds to wait=w25) -> ()  [unwired: 1 out]
      }
    }
  }
